vi "Determine Warning_Ex 4-1.vi"(8 "error in (no error)":errorcluster, 9 "Min Temp":dbl, 10 "Max Temp":dbl, 11 "Current Temp":dbl) -> (0 "error out":errorcluster, 1 "Warning?":bool, 2 "Warning Text":string)   [LabVIEW 2014]
doc: "This VI is an exercise in the LabVIEW Core I course. During this exercise, you modify the code to use a Formula Node and/or a Case structure."
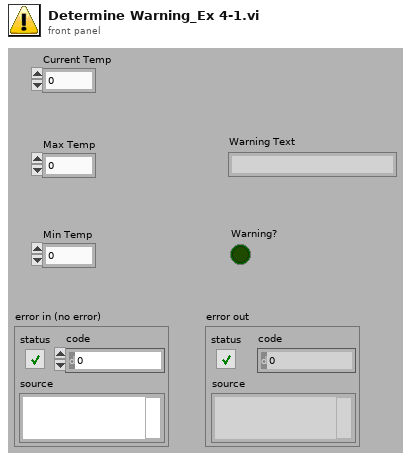
[diagram p1: front panel]
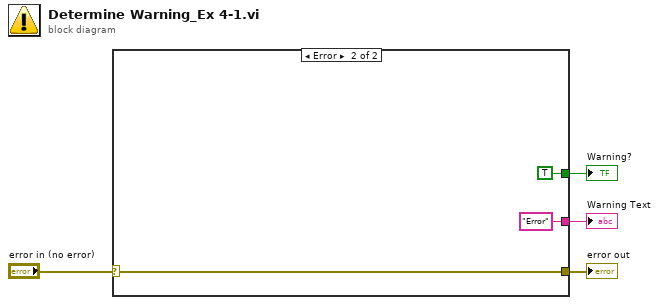
[diagram p0: block diagram]
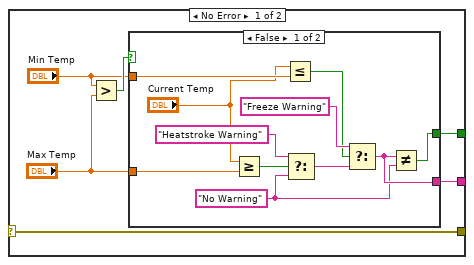
[diagram p2: hidden frame]
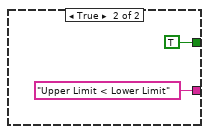
[diagram p3: hidden frame]
diagram:
  n1 = case shown="Error" "error in (no error)" {
    selector: "error in (no error)" -> [w5 w26]
    tunnel: [w7 TRUE] -> w3
    tunnel: [w6 "Error" ("f")] -> w2
    tunnel: [w5 w26] -> w1
    frame No Error {
      n2 = Greater?(x="Min Temp", y="Max Temp") -> (0:w10:bool)
      n3 = case shown="False" w10 {
        tunnel: [w21 "Upper Limit < Lower Limit" ("f")] -> w6
        tunnel: [w20 TRUE] -> w7
        tunnel: "Max Temp" -> [w19 _]
        tunnel: "Min Temp" -> [w16 _]
        frame False {
          w11 = "No Warning" ("f")
          n4 = Greater Or Equal?(x="Current Temp", y=w19) -> (x >= y?=w18:bool)
          n5 = Less Or Equal?(x="Current Temp", y=w16) -> (x <= y?=w13:bool)
          n6 = Select(t="Heatstroke Warning", s=w18, f=w11) -> (s? t:f=w12:string)
          n7 = Select(t="Freeze Warning", s=w13, f=w12) -> (s? t:f=w21:string)
          n8 = Not Equal?(x=w21, y=w11) -> (x != y?=w20:bool)
        }
        frame True {
        }
      }
    }
    frame Error {
    }
  }
  "error out" <- w1
  "Warning?" <- w3
  "Warning Text" <- w2
